vi "Save Digital Data.vi"(8 "error in (no error)":errorcluster, 10 "Data Cluster":cluster{"Path":path, "Array":bool[]}, 11 "Digital Logging in":refnum<class "Digital Logging.lvclass">) -> (0 "error out":errorcluster, 3 "Digital Logging out":refnum<class "Digital Logging.lvclass">)   [LabVIEW 2020, in "Digital Logging.lvlib" / "Digital Logging.lvclass"]
uses:
  Digital Logging.lvclass
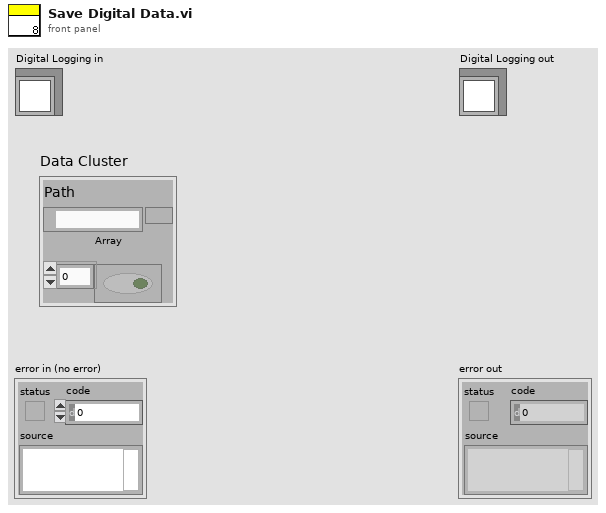
[diagram p1: front panel]
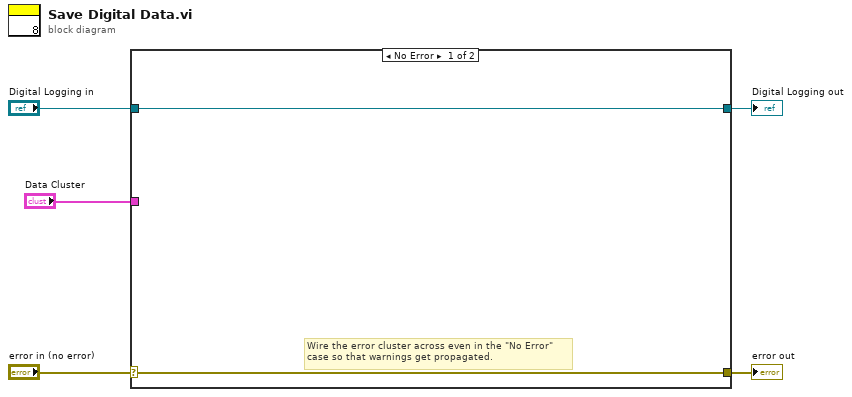
[diagram p0: block diagram]
diagram:
  n1 = case shown="No Error" "error in (no error)" {
    selector: "error in (no error)" -> [w6 w9]
    tunnel: [w6 w9] -> w4
    tunnel: [w7 w8] -> w2
    tunnel: "Digital Logging in" -> [w7 w8]
    tunnel: "Data Cluster" -> [_ _]
    frame No Error {
      # "Wire the error cluster across even in the \"No Error\"\ncase so that warnings get propagated."
    }
    frame Error {
    }
  }
  "error out" <- w4
  "Digital Logging out" <- w2
